vi "Check If Pixels Belong In SectorV2.vi"() -> (3 "FIFO Timeout?":bool)   [LabVIEW 2013]
uses:
  Single Sector Pixel Cluster.ctl
  Globals/Sector Parameter Global.vi
  Globals/Pixel Location Global.vi
  <vilib>/rvi/FIFO/Fifo_Resource/nirvififoEmulationReadFpgaImpl.vi
  <vilib>/rvi/DataTransferAndStorage/Container/Common/niFpgaContainerGetUniqueNameForEmu.vi
  <vilib>/rvi/FIFO/Fifo_Resource/nirvififoEmulationWriteFpgaImpl.vi
  <vilib>/rvi/DataTransferAndStorage/Container/XNode/niFpgaContainer.xnode
  <vilib>/rvi/FIFO/Fifo_Resource/nirvififoEmulationRead.vi
  <vilib>/rvi/FIFO/Fifo_Resource/nirvififoEmulationWrite.vi
panel:
  out "End of  Data?":bool
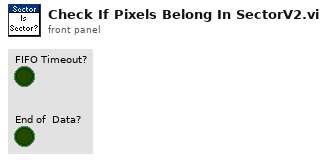
[diagram p1: front panel]
types:
  T1 = typedef "Single Sector Pixel Cluster.ctl" = cluster{"Sector #":u8, "Pixel Value":u8}
  T2 = typedef "Sector Parameter Cluster.ctl" = cluster{"Start Angle":fxp<+/-,17,2>, "End Angle":fxp<+,17,3>, "Inner Radius":u16, "Outter Radius":u16, "Hinge X":u16, "Hinge Y":u16, "NumWingSectors":u8}
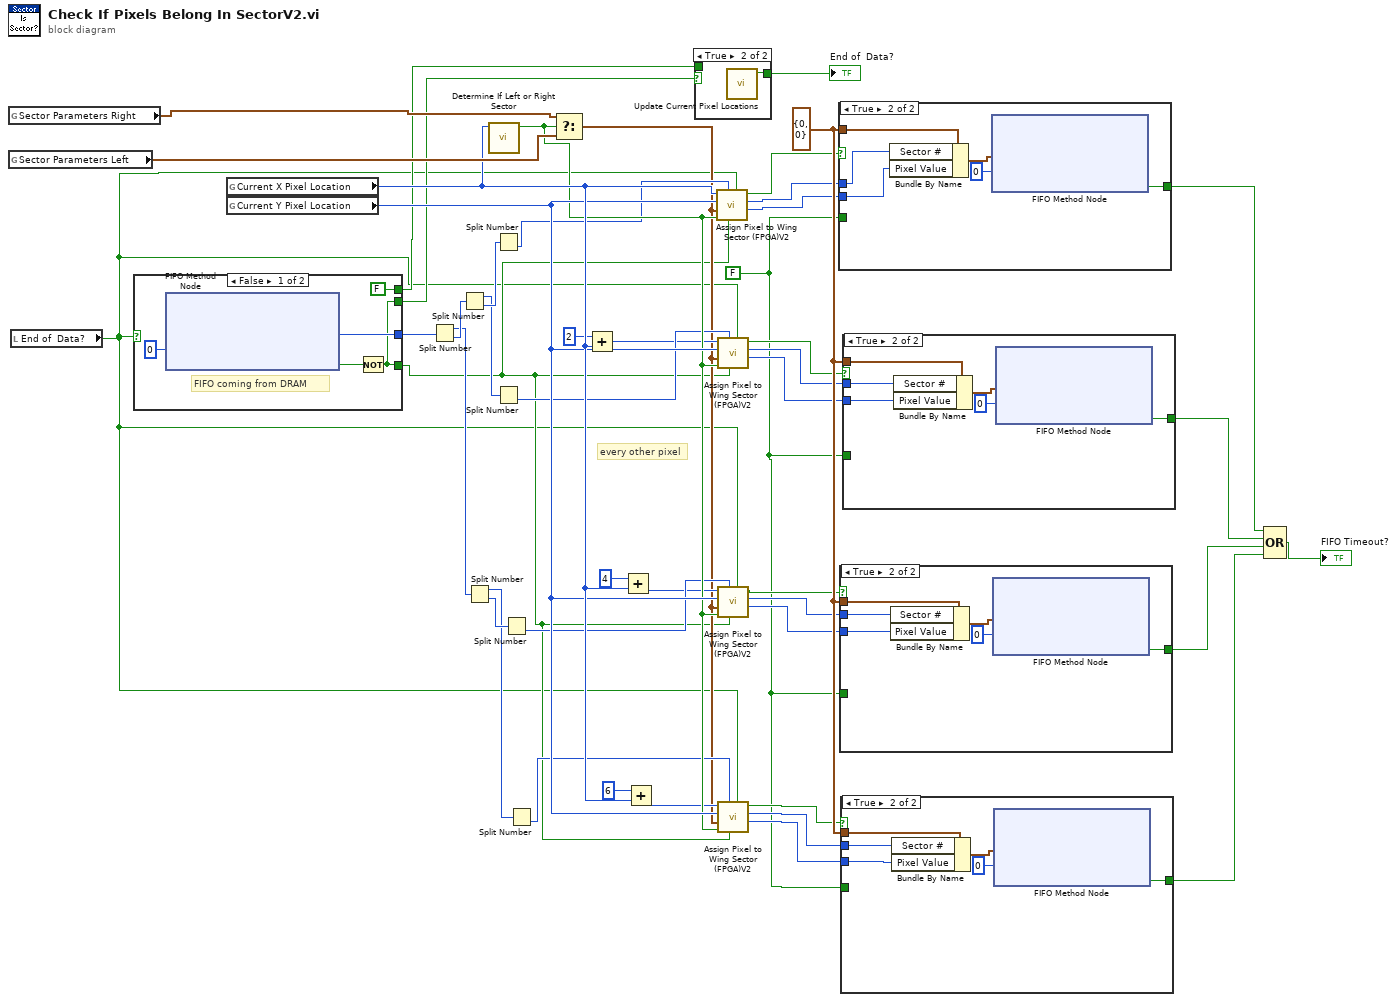
[diagram p0: block diagram]
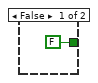
[diagram p3: hidden frame]
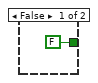
[diagram p4: hidden frame]
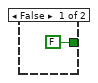
[diagram p5: hidden frame]
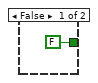
[diagram p6: hidden frame]
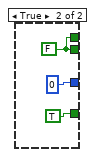
[diagram p7: hidden frame]
diagram:
  w23 = FALSE
  w36 = T1 {"Sector #"=0, "Pixel Value"=0} ("Single Sector Pixel")
  # "every other pixel"
  n1 = global read "Sector Parameter Global.vi" "Sector Parameters Right"() -> (w45:T2)
  n2 = global read "Sector Parameter Global.vi" "Sector Parameters Left"() -> (w44:T2)
  n3 = local read "End of  Data?"() -> (w1:bool)
  n4 = case shown="False" w1 {
    tunnel: [w49 TRUE ("Timed Out?")] -> w4
    tunnel: [w51 u64 0 ("Element")] -> w41
    tunnel: [w49 w53] -> w3
    tunnel: [FALSE ("Timed Out?") w53] -> w2
    frame False {
      # "FIFO coming from DRAM"
      n5 = xnode ("FIFO Method Node")("Timeout"=0) -> ("Element"=w51:u64, "Timed Out?"=w50:bool)  [unwired: 1 in, 1 out]
      n6 = Not(x=w50) -> (.not. x?=w49:bool)
    }
    frame True {
      w53 = FALSE ("Timed Out?")
    }
  }
  n7 = global read "Pixel Location Global.vi" "Current X Pixel Location"() -> (w43:u16)
  n8 = global read "Pixel Location Global.vi" "Current Y Pixel Location"() -> (w42:u16)
  n9 = Split Number(x=w41) -> (hi(x)=w21:u32, lo(x)=w22:u32)
  n10 = Split Number(x=w22) -> (hi(x)=w19:u16, lo(x)=w20:u16)
  n11 = Split Number(x=w21) -> (hi(x)=w17:u16, lo(x)=w18:u16)
  n12 = call "Determine If Left or Right Sector.vi"("X Pixel Location"=w43) -> ("Right Sector?"=w16:bool)  [unwired: 10 in]
  n13 = Split Number(x=w20) -> (lo(x)=w15:u8)  [unwired: 1 out]
  n14 = Split Number(x=w19) -> (lo(x)=w14:u8)  [unwired: 1 out]
  n15 = Split Number(x=w18) -> (lo(x)=w13:u8)  [unwired: 1 out]
  n16 = Split Number(x=w17) -> (lo(x)=w12:u8)  [unwired: 1 out]
  n17 = Select(t=w45, s=w16, f=w44) -> (s? t:f=w5:T2)
  n18 = Add(x=u16 2, y=w43) -> (x+y=w8:u16)
  n19 = Add(x=u16 4, y=w43) -> (x+y=w7:u16)
  n20 = Add(x=u16 6, y=w43) -> (x+y=w6:u16)
  n21 = case shown="True" w3 {
    tunnel: [w56 w57] -> w47
    tunnel: w2 -> [w56 _]
    frame False {
    }
    frame True {
      n22 = call "Update Current Pixel Locations.vi"() -> ("End of data?"=w57:bool)  [unwired: 11 in]
    }
  }
  "End of  Data?" <- w47
  n23 = call "Assign Pixel to Wing Sector (FPGA)V2.vi"("End of Data?"=w1, "Valid Data?"=w4, "Pixel Intensity In"=w15, "Right Wing?"=w16, "Sector Parameters"=w5, "Pixel Y"=w42, "Pixel X"=w43) -> ("Pixel Intensity Out"=w33:u8, "sector #"=w34:u8, "output valid"=w35:bool)  [unwired: 1 in]
  n24 = call "Assign Pixel to Wing Sector (FPGA)V2.vi"("End of Data?"=w1, "Valid Data?"=w4, "Pixel Intensity In"=w14, "Right Wing?"=w16, "Sector Parameters"=w5, "Pixel Y"=w42, "Pixel X"=w8) -> ("Pixel Intensity Out"=w30:u8, "sector #"=w31:u8, "output valid"=w32:bool)  [unwired: 1 in]
  n25 = call "Assign Pixel to Wing Sector (FPGA)V2.vi"("End of Data?"=w1, "Valid Data?"=w4, "Pixel Intensity In"=w13, "Right Wing?"=w16, "Sector Parameters"=w5, "Pixel Y"=w42, "Pixel X"=w7) -> ("Pixel Intensity Out"=w27:u8, "sector #"=w28:u8, "output valid"=w29:bool)  [unwired: 1 in]
  n26 = call "Assign Pixel to Wing Sector (FPGA)V2.vi"("End of Data?"=w1, "Valid Data?"=w4, "Pixel Intensity In"=w12, "Right Wing?"=w16, "Sector Parameters"=w5, "Pixel Y"=w42, "Pixel X"=w6) -> ("Pixel Intensity Out"=w24:u8, "sector #"=w25:u8, "output valid"=w26:bool)  [unwired: 1 in]
  n27 = case shown="True" w35 {
    tunnel: w36 -> [_ w59]
    tunnel: [FALSE ("Timed Out?") w62] -> w40
    tunnel: w34 -> [_ w60]
    tunnel: w33 -> [_ w61]
    tunnel: w23 -> [_ _]
    frame False {
    }
    frame True {
      n28 = Bundle By Name(cluster=w59, "Sector #"=w60, "Pixel Value"=w61) -> (w63:T1)
      n29 = xnode ("FIFO Method Node")("Element"=w63, "Timeout"=0) -> ("Timed Out?"=w62:bool)  [unwired: 1 in, 1 out]
    }
  }
  n30 = case shown="True" w29 {
    tunnel: w36 -> [_ w71]
    tunnel: [FALSE ("Timed Out?") w68] -> w38
    tunnel: w28 -> [_ w66]
    tunnel: w27 -> [_ w67]
    tunnel: w23 -> [_ _]
    frame False {
    }
    frame True {
      n31 = Bundle By Name(cluster=w71, "Sector #"=w66, "Pixel Value"=w67) -> (w69:T1)
      n32 = xnode ("FIFO Method Node")("Element"=w69, "Timeout"=0) -> ("Timed Out?"=w68:bool)  [unwired: 1 in, 1 out]
    }
  }
  n33 = case shown="True" w26 {
    tunnel: w36 -> [_ w78]
    tunnel: [FALSE ("Timed Out?") w75] -> w37
    tunnel: w25 -> [_ w73]
    tunnel: w24 -> [_ w74]
    tunnel: w23 -> [_ _]
    frame False {
    }
    frame True {
      n34 = Bundle By Name(cluster=w78, "Sector #"=w73, "Pixel Value"=w74) -> (w76:T1)
      n35 = xnode ("FIFO Method Node")("Element"=w76, "Timeout"=0) -> ("Timed Out?"=w75:bool)  [unwired: 1 in, 1 out]
    }
  }
  n36 = case shown="True" w32 {
    tunnel: w36 -> [_ w85]
    tunnel: [FALSE ("Timed Out?") w82] -> w39
    tunnel: w31 -> [_ w80]
    tunnel: w30 -> [_ w81]
    tunnel: w23 -> [_ _]
    frame False {
    }
    frame True {
      n37 = Bundle By Name(cluster=w85, "Sector #"=w80, "Pixel Value"=w81) -> (w83:T1)
      n38 = xnode ("FIFO Method Node")("Element"=w83, "Timeout"=0) -> ("Timed Out?"=w82:bool)  [unwired: 1 in, 1 out]
    }
  }
  n39 = Compound Arithmetic op=OR(w40, w39, w38, w37) -> (→"FIFO Timeout?":bool)
